vi "Sample Rate To Loop Time (ms).vi"(0 "sample rate (S/s)":dbl format="%#_6p", 1 "FPGA clock rate (Hz)":dbl=40000000.0 format="%#_6p", 11 "error in (no error)":errorcluster) -> (4 "count (ms/S)":u32, 10 "actual sample rate (S/s)":dbl format="%#_6p", 15 "error out":errorcluster)   [LabVIEW 2020, in "NI_FpgaMspHost.lvlib"]
doc: "Converts the desired sample rate to the appropriate count for the Loop Timer Express VI and computes the achievable sample rate for use with other Scaling VIs."
uses:
  <vilib>/rvi/Analysis/host/Public/NI_FpgaMspHost.lvlib
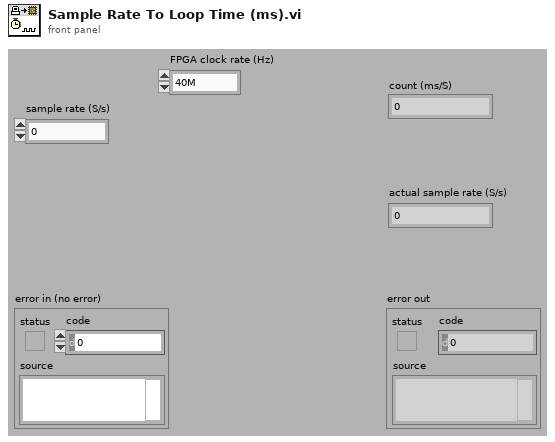
[diagram p1: front panel]
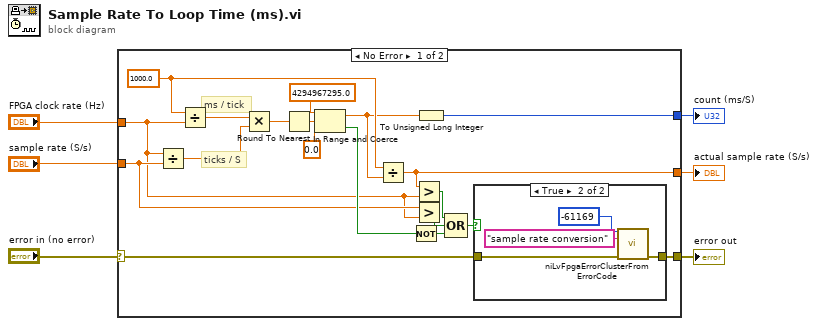
[diagram p0: block diagram]
diagram:
  n1 = case shown="No Error" "error in (no error)" {
    selector: "error in (no error)" -> [w22 w31]
    tunnel: "FPGA clock rate (Hz)" -> [w11 _]
    tunnel: "sample rate (S/s)" -> [w12 _]
    tunnel: [w21 _] -> w1
    tunnel: [w13 _] -> w3
    tunnel: [w23 w31] -> w2
    frame No Error {
      w19 = 1000.0 ("x")
      # "ticks / S"
      # "ms / tick"
      n2 = Divide(x=w11, y=w12) -> (x/y=w24:dbl)
      n3 = Divide(x=w19, y=w11) -> (x/y=w25:dbl)
      n4 = Multiply(x=w25, y=w24) -> (x*y=w8:dbl)
      n5 = Round To Nearest(number=w8) -> (nearest integer value=w7:dbl)
      n6 = In Range and Coerce(upper limit=4294967295.0 ("unsigned 32bit integer"), x=w7, lower limit=0.0) -> (coerced(x)=w9:dbl, In Range?=w16:bool)
      n7 = Divide(x=w19, y=w9) -> (x/y=w13:dbl)
      n8 = Not(x=w16) -> (.not. x?=w14:bool)
      n9 = Greater?(x=w13, y=w11) -> (0:w15:bool)
      n10 = Greater?(x=w12, y=w11) -> (0:w10:bool)
      n11 = To Unsigned Long Integer(number=w9) -> (unsigned 32bit integer=w21:u32)
      n12 = Compound Arithmetic op=OR(w15, w10, w14) -> (w20:bool)
      n13 = case shown="True" w20 {
        tunnel: [w26 w30] -> w23
        tunnel: w22 -> [w26 w27]
        frame False {
        }
        frame True {
          n14 = call <vilib>:"niLvFpgaErrorClusterFromErrorCode.vi"("error code"=-61169, "function name"="sample rate conversion" ("L10N_Function Name"), "error in"=w27) -> ("error out"=w30:errorcluster)  [unwired: 4 in, 8 out]
        }
      }
    }
    frame Error {
    }
  }
  "error out" <- w2
  "count (ms/S)" <- w1
  "actual sample rate (S/s)" <- w3
